vi "PQresultStatus.vi"(8 "error in (no error)":errorcluster, 10 "res":u32) -> (0 "error out":errorcluster, 1 "PQresultStatus":T1(ring), 2 "res out":u32)   [LabVIEW 2019, in "libpqlv.lvlib"]
doc: "Returns the result status of the command."
uses:
  libpqlv.lvlib
  libpq.dll
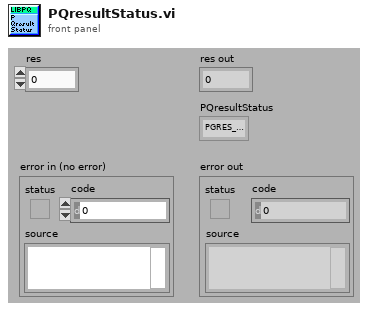
[diagram p1: front panel]
types:
  T1 = enum32{"PGRES_EMPTY_QUERY", "PGRES_COMMAND_OK", "PGRES_TUPLES_OK", "PGRES_COPY_OUT", "PGRES_COPY_IN", "PGRES_BAD_RESPONSE", "PGRES_NONFATAL_ERROR", "PGRES_FATAL_ERROR"}
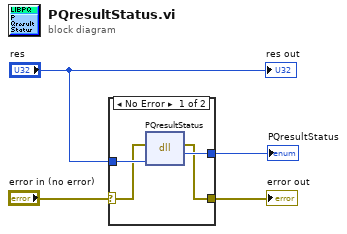
[diagram p0: block diagram]
diagram:
  n1 = case shown="No Error" "error in (no error)" {
    selector: "error in (no error)" -> [w6 w9]
    tunnel: [w5 w9] -> w3
    tunnel: [w8 _] -> w2
    tunnel: "res" -> [w7 _]
    frame No Error {
      n2 = dll-call lib="libpq.*" fn="PQresultStatus"(error in=w6, "res"=w7) -> (error out=w5:errorcluster, "PQresultStatus"=w8:u32)  [unwired: 3 in, 1 out]
    }
    frame Error {
    }
  }
  "error out" <- w3
  "PQresultStatus" <- w2
  "res out" <- "res"
